vi "DataLog Read Log Time Range.vi"(0 "tag log directory":path, 5 "begin of range":dbl format="%<%H:%M:%S%2u\n%Y/%m/%d>T", 9 "end of range":dbl format="%<%H:%M:%S%2u\n%Y/%m/%d>T", 11 "error in (no error)":errorcluster) -> (4 "dup tag log directory":path, 6 "too many points?":bool, 8 "time range of points":T1[](array[typedef]) {"value" format="%.3e"; "time" format="%<%H:%M:%S%2u\n%Y/%m/%d>T"}, 15 "error out":errorcluster)   [LabVIEW 2012]
doc: "Read a range of points that covers the specified time range from a tag's log. The first returned point's time <= begin, the last returned point's time >= end. An exception to this rule occurs when the range begins before the oldest point in the log or ends after the last point in the log. In that case as much data as possible will be returned. If the range lies before the logged data, only the first point will be returned. If the range lies beyond the logged data, only the last point will be returned."
uses:
  typedefs/clusters/t_DataLog Point.ctl
  private/glb_DataLog MCVD.vi
  private/glb_DataLog Runtime Parameterisation.vi
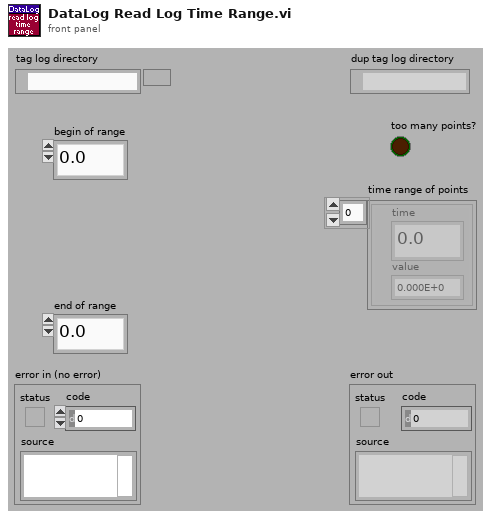
[diagram p1: front panel]
types:
  T1 = typedef "t_DataLog Point.ctl" = cluster{"time":dbl, "value":dbl}
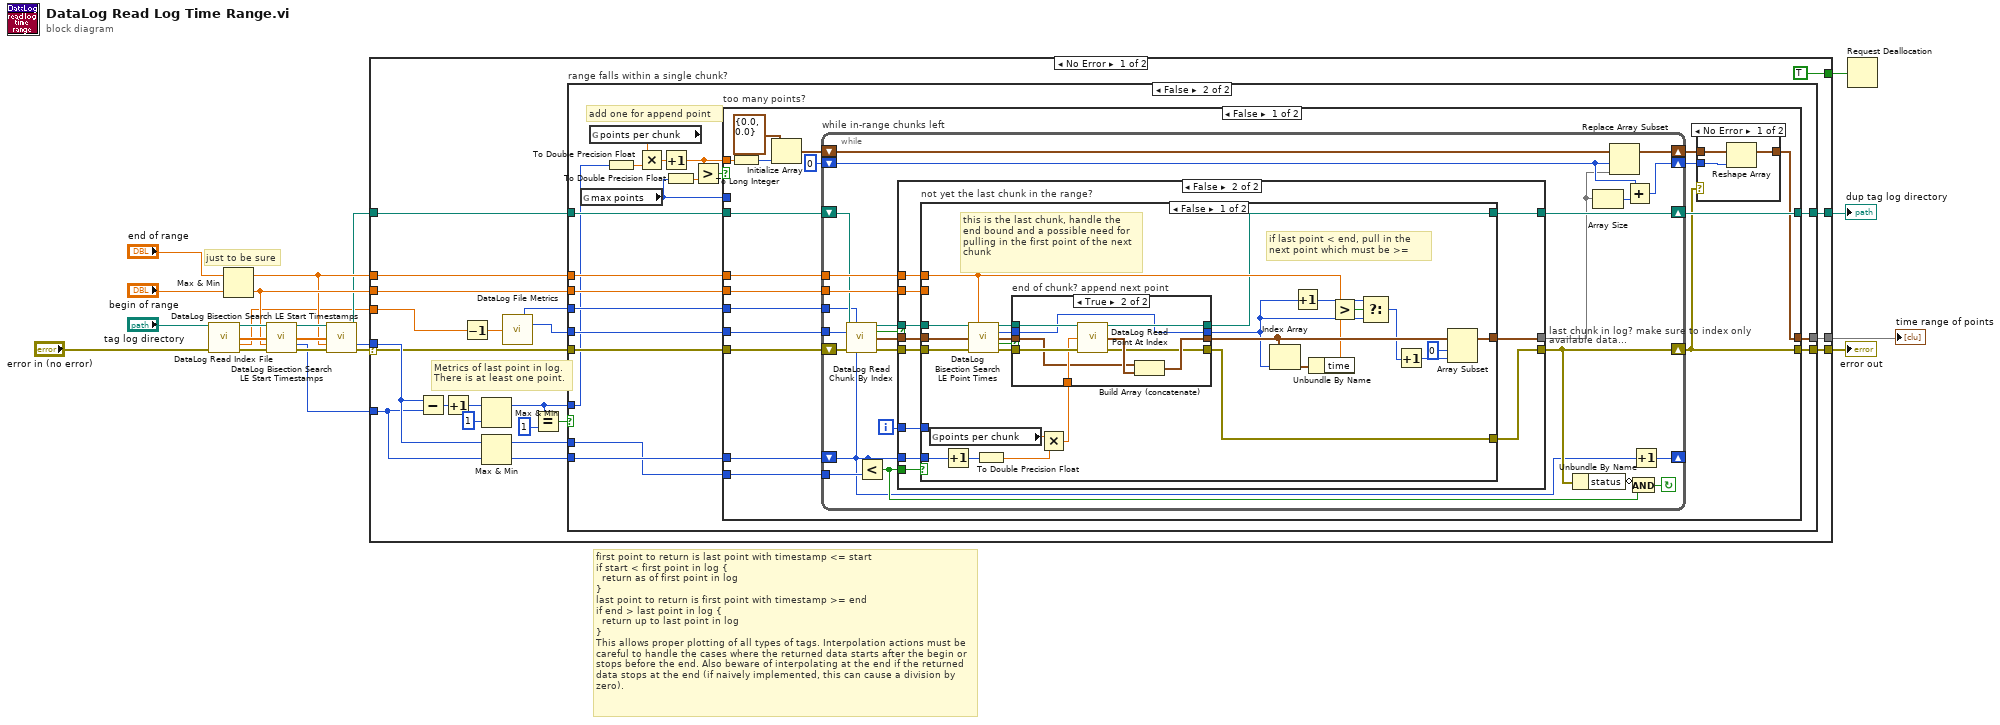
[diagram p0: block diagram]
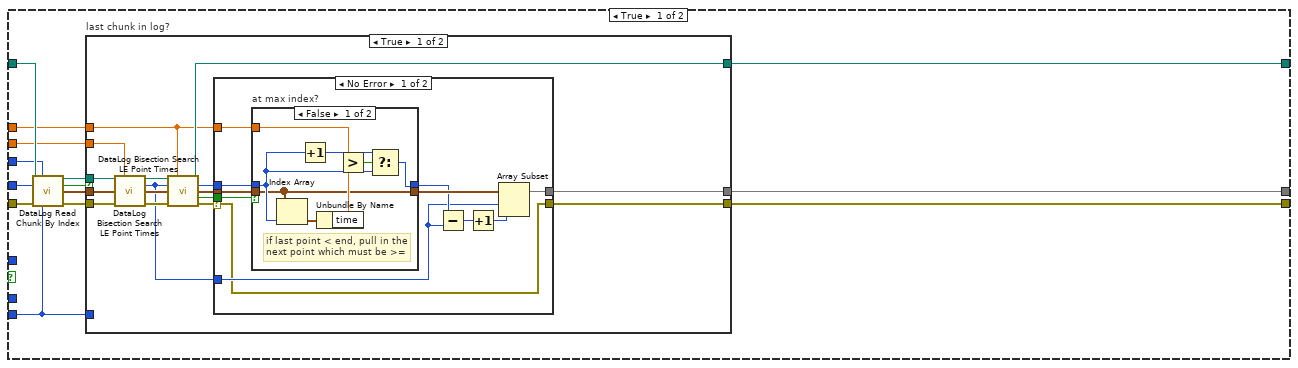
[diagram p2: hidden frame]
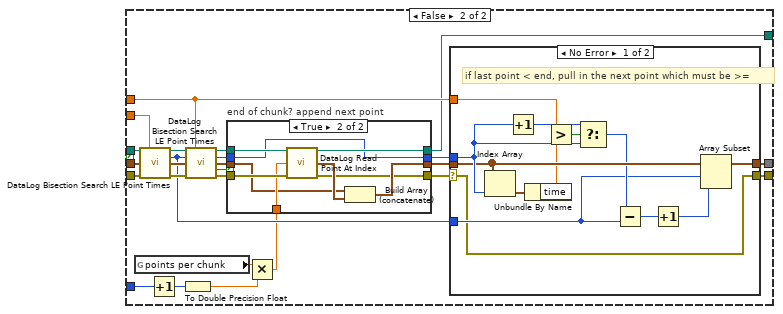
[diagram p5: hidden frame]
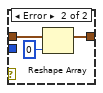
[diagram p8: hidden frame]
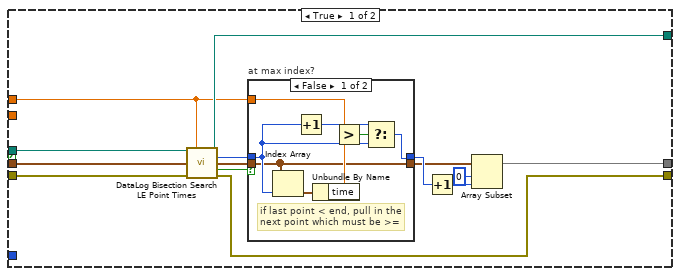
[diagram p9: hidden frame]
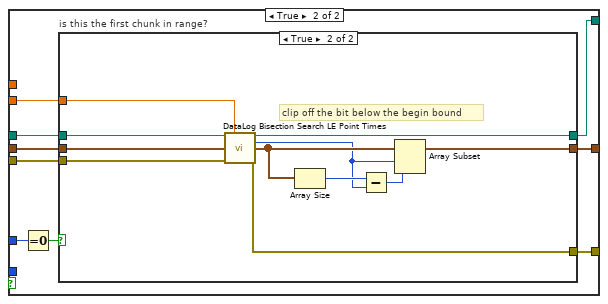
[diagram p12: hidden frame]
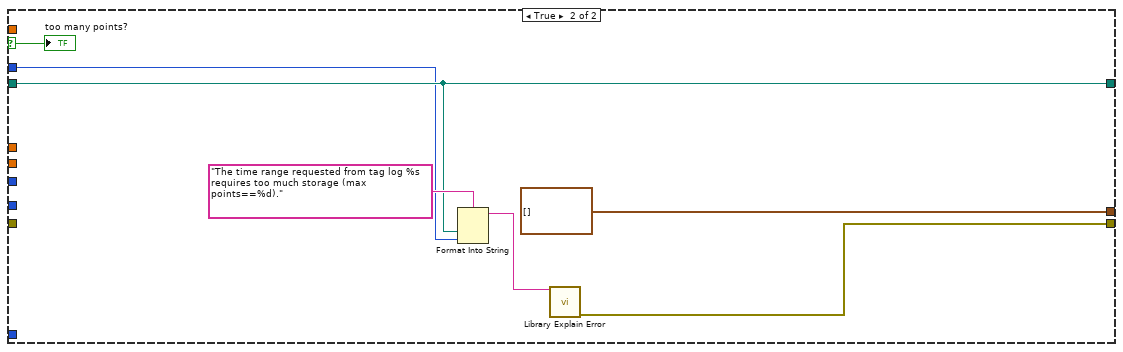
[diagram p14: hidden frame]
diagram:
  # "just to be sure"
  # "first point to return is last point with timestamp <= start\nif start < first point in log {\n  return as of first point in log\n}\nlast point to return is first point with timestamp >= end\nif end > last point in log {\n  return up to last point in log\n}\nThis allows proper plotting of all types of tags. Interpolation actions must be careful to handle the cases where the returned data starts after the begin or stops before the end. Also beware of interpolating at the end if the returned data stops at the end (if naively implemented, this can cause a division by zero)."
  n1 = call "DataLog Read Index File.vi"("tag log directory"="tag log directory", "error in (no error)"="error in (no error)") -> ("dup tag log directory"=w13:path, "chunk start timestamps"=w14:dbl[], "write index"=w4:dbl, "error out"=w12:errorcluster)  [unwired: 10 in]
  n2 = Max & Min(x="end of range", y="begin of range") -> (max(x,y)=w6:dbl, min(x,y)=w7:dbl)
  n3 = call "DataLog Bisection Search LE Start Timestamps.vi"("tag log directory"=w13, "chunk start timestamps"=w14, "search timestamp"=w7, "error in (no error)"=w12) -> ("dup tag log directory"=w11:path, "dup chunk start timestamps"=w10:dbl[], "nearest chunk index"=w3:i32, "error out"=w9:errorcluster)  [unwired: 8 in]
  n4 = call "DataLog Bisection Search LE Start Timestamps.vi"("tag log directory"=w11, "chunk start timestamps"=w10, "search timestamp"=w6, "error in (no error)"=w9) -> ("dup tag log directory"=w5:path, "nearest chunk index"=w8:i32, "error out"=w2:errorcluster)  [unwired: 8 in, 1 out]
  n5 = case shown="No Error" w2 {
    selector: w2 -> [w23 w320]
    tunnel: [w43 w320] -> w21
    tunnel: [w42 w321] -> w18
    tunnel: [w41 _] -> w17
    tunnel: w8 -> [w38 _]
    tunnel: w7 -> [w33 _]
    tunnel: w6 -> [w32 _]
    tunnel: w5 -> [w30 w321]
    tunnel: w4 -> [w27 _]
    tunnel: w3 -> [w24 _]
    tunnel: [TRUE _] -> w1
    frame No Error {
      # "Metrics of last point in log.\nThere is at least one point."
      n6 = Subtract(x=w38, y=w24) -> (x-y=w40:i32)
      n7 = Increment(x=w40) -> (x+1=w34:i32)
      n8 = Decrement(x=w27) -> (x-1=w28:dbl)
      n9 = Max & Min(x=w34, y=1) -> (max(x,y)=w25:i32)  [unwired: 1 out]
      n10 = Max & Min(x=w38, y=w24) -> (max(x,y)=w31:i32, min(x,y)=w37:i32)
      n11 = call "DataLog File Metrics.vi"("point index"=w28) -> ("index in chunk"=w26:i32, "chunk index"=w29:i32)  [unwired: 9 in, 4 out]
      n12 = Equal?(x=w25, y=1) -> (x = y?=w35:bool)
      n13 = case "range falls within a single chunk?" shown="False" w35 {
        tunnel: w30 -> [w57 w161]
        tunnel: w23 -> [w56 w159]
        tunnel: w37 -> [w45 w162]
        tunnel: w33 -> [w51 w166]
        tunnel: w32 -> [w50 w165]
        tunnel: [w52 w154] -> w43
        tunnel: [w49 w160] -> w42
        tunnel: w31 -> [_ w155]
        tunnel: w29 -> [w46 w163]
        tunnel: w26 -> [w44 w164]
        tunnel: [w48 w153] -> w41
        tunnel: w25 -> [_ w158]
        frame True {
          n14 = call "DataLog Read Chunk By Index.vi"("tag log directory"=w57, "index in last chunk"=w44, "index of last chunk"=w46, "error in (no error)"=w56, "chunk index"=w45) -> ("dup tag log directory"=w53:path, "last chunk in log?"=w47:bool, "chunk of points"=w54:T1[], "error out"=w55:errorcluster)  [unwired: 7 in]
          n15 = case "last chunk in log?" shown="True" w47 {
            tunnel: w55 -> [w73 w120]
            tunnel: w54 -> [w72 w119]
            tunnel: w53 -> [w68 w115]
            tunnel: [w62 w111] -> w52
            tunnel: w51 -> [w66 w114]
            tunnel: w50 -> [w59 w112]
            tunnel: [w65 w102] -> w49
            tunnel: [w63 w110] -> w48
            tunnel: w45 -> [_ w96]
            frame True {
              n16 = call "DataLog Bisection Search LE Point Times.vi"("tag log directory"=w68, "search timestamp"=w66, "points"=w72, "error in (no error)"=w73) -> ("dup tag log directory"=w69:path, "index"=w58:i32, "dup points"=w71:T1[], "error out"=w70:errorcluster)  [unwired: 7 in, 1 out]
              n17 = call "DataLog Bisection Search LE Point Times.vi"("tag log directory"=w69, "search timestamp"=w59, "min index (0)"=w58, "points"=w71, "error in (no error)"=w70) -> ("dup tag log directory"=w65:path, "index"=w61:i32, "dup points"=w67:T1[], "at max?"=w60:bool, "error out"=w64:errorcluster)  [unwired: 6 in]
              n18 = case shown="No Error" w64 {
                selector: w64 -> [w74 w95]
                tunnel: w67 -> [w82 _]
                tunnel: [w79 _] -> w63
                tunnel: [w74 w95] -> w62
                tunnel: w61 -> [w83 _]
                tunnel: w60 -> [w84 _]
                tunnel: w59 -> [w81 _]
                tunnel: w58 -> [w77 _]
                frame No Error {
                  n19 = case "at max index?" shown="False" w84 {
                    tunnel: w83 -> [w87 w94]
                    tunnel: [w86 w94] -> w78
                    tunnel: [w85 w93] -> w80
                    tunnel: w82 -> [w85 w93]
                    tunnel: w81 -> [w91 _]
                    frame False {
                      # "if last point < end, pull in the next point which must be >="
                      n20 = Index Array(array=w85, index=w87) -> (element=w92:T1)
                      n21 = Increment(x=w87) -> (x+1=w88:i32)
                      n22 = Unbundle By Name(w92) -> ("time"=w90:dbl)
                      n23 = Greater?(x=w91, y=w90) -> (0:w89:bool)
                      n24 = Select(t=w88, s=w89, f=w87) -> (s? t:f=w86:i32)
                    }
                    frame True {
                    }
                  }
                  n25 = Subtract(x=w78, y=w77) -> (x-y=w76:i32)
                  n26 = Increment(x=w76) -> (x+1=w75:i32)
                  n27 = Array Subset(array=w80, index=w77, length=w75) -> (w79:T1[])
                }
                frame Error {
                }
              }
            }
            frame False {
              n28 = global read "glb_DataLog MCVD.vi" "points per chunk"() -> (w100:dbl)
              n29 = call "DataLog Bisection Search LE Point Times.vi"("tag log directory"=w115, "search timestamp"=w114, "points"=w119, "error in (no error)"=w120) -> ("dup tag log directory"=w116:path, "index"=w113:i32, "dup points"=w118:T1[], "error out"=w117:errorcluster)  [unwired: 7 in, 1 out]
              n30 = Increment(x=w96) -> (x+1=w97:i32)
              n31 = To Double Precision Float(number=w97) -> (double precision float=w99:dbl)
              n32 = call "DataLog Bisection Search LE Point Times.vi"("tag log directory"=w116, "search timestamp"=w112, "min index (0)"=w113, "points"=w118, "error in (no error)"=w117) -> ("dup tag log directory"=w107:path, "index"=w103:i32, "dup points"=w106:T1[], "at max?"=w109:bool, "error out"=w108:errorcluster)  [unwired: 6 in]
              n33 = Multiply(x=w100, y=w99) -> (x*y=w98:dbl)
              n34 = case "end of chunk? append next point" shown="True" w109 {
                tunnel: w108 -> [w121 w133]
                tunnel: w107 -> [w122 w131]
                tunnel: [w124 w128] -> w105
                tunnel: w106 -> [w124 w129]
                tunnel: w103 -> [w123 w125]
                tunnel: [w123 w125] -> w104
                tunnel: [w122 w127] -> w102
                tunnel: [w121 w126] -> w101
                tunnel: w98 -> [_ w132]
                frame False {
                }
                frame True {
                  n35 = call "DataLog Read Point At Index.vi"("tag log directory"=w131, "log index"=w132, "error in (no error)"=w133) -> ("dup tag log directory"=w127:path, "point"=w130:T1, "error out"=w126:errorcluster)  [unwired: 10 in]
                  n36 = Build Array (concatenate)(w129, w130) -> (w128:T1[])
                }
              }
              n37 = case shown="No Error" w101 {
                selector: w101 -> [w134 w147]
                tunnel: w105 -> [w145 _]
                tunnel: [w143 _] -> w110
                tunnel: [w134 w147] -> w111
                tunnel: w104 -> [w146 _]
                tunnel: w112 -> [w144 _]
                tunnel: w113 -> [w141 _]
                frame No Error {
                  # "if last point < end, pull in the next point which must be >="
                  n38 = Index Array(array=w145, index=w146) -> (element=w140:T1)
                  n39 = Increment(x=w146) -> (x+1=w137:i32)
                  n40 = Unbundle By Name(w140) -> ("time"=w139:dbl)
                  n41 = Greater?(x=w144, y=w139) -> (0:w138:bool)
                  n42 = Select(t=w137, s=w138, f=w146) -> (s? t:f=w142:i32)
                  n43 = Subtract(x=w142, y=w141) -> (x-y=w136:i32)
                  n44 = Increment(x=w136) -> (x+1=w135:i32)
                  n45 = Array Subset(array=w145, index=w141, length=w135) -> (w143:T1[])
                }
                frame Error {
                }
              }
            }
          }
        }
        frame False {
          # "add one for append point"
          n46 = global read "glb_DataLog Runtime Parameterisation.vi" "max points"() -> (w148:i32)
          n47 = global read "glb_DataLog MCVD.vi" "points per chunk"() -> (w156:dbl)
          n48 = To Double Precision Float(number=w158) -> (double precision float=w157:dbl)
          n49 = Multiply(x=w156, y=w157) -> (x*y=w151:dbl)
          n50 = Increment(x=w151) -> (x+1=w150:dbl)
          n51 = To Double Precision Float(number=w148) -> (double precision float=w149:dbl)
          n52 = Greater?(x=w150, y=w149) -> (0:w152:bool)
          n53 = case "too many points?" shown="False" w152 {
            selector: w152 -> [_ w313]
            tunnel: w166 -> [w184 _]
            tunnel: w165 -> [w183 _]
            tunnel: w164 -> [w182 _]
            tunnel: w163 -> [w181 _]
            tunnel: w162 -> [w180 _]
            tunnel: w161 -> [w179 w315]
            tunnel: [w178 w315] -> w160
            tunnel: w159 -> [w177 _]
            tunnel: [w169 T1[] []] -> w153
            tunnel: [w168 w318] -> w154
            tunnel: w155 -> [w176 _]
            tunnel: w150 -> [w175 _]
            tunnel: w148 -> [_ w314]
            frame False {
              n54 = To Long Integer(number=w175) -> (32bit integer=w174:i32)
              n55 = Initialize Array(T1 {"time"=0.0, "value"=0.0} ("point"), w174) -> (w167:T1[])
              n56 = while "while in-range chunks left" {
                tunnel: w184 -> [w212]
                tunnel: w183 -> [w211]
                tunnel: w182 -> [w195]
                tunnel: w181 -> [w193]
                shift-right: [w207] -> _
                shift-left: w180 -> [w194]
                shift-right: [w209] -> w178
                shift-left: w179 -> [w210]
                shift-right: [w196] -> w171
                shift-left: w167 -> [w203]
                shift-right: [w205] -> w168
                shift-left: w177 -> [w208]
                tunnel: w176 -> [w206]
                shift-right: [w201] -> w170
                shift-left: 0 -> [w202]
                i -> [w198]
                stop <- w204 continue-if-true
                n57 = call "DataLog Read Chunk By Index.vi"("tag log directory"=w210, "index in last chunk"=w195, "index of last chunk"=w193, "error in (no error)"=w208, "chunk index"=w194) -> ("dup tag log directory"=w213:path, "last chunk in log?"=w192:bool, "chunk of points"=w214:T1[], "error out"=w215:errorcluster)  [unwired: 7 in]
                n58 = Less?(x=w194, y=w206) -> (x < y?=w199:bool)
                n59 = case "last chunk in log? make sure to index only available data..." shown="False" w192 {
                  tunnel: w215 -> [w221 w244]
                  tunnel: w214 -> [w222 w245]
                  tunnel: w213 -> [w223 w243]
                  tunnel: [w216 w249] -> w205
                  tunnel: w212 -> [_ w240]
                  tunnel: w211 -> [w224 w250]
                  tunnel: [w228 w247] -> w209
                  tunnel: [w227 w248] -> w191
                  tunnel: w194 -> [_ w246]
                  tunnel: w199 -> [_ w242]
                  tunnel: w198 -> [_ w241]
                  frame True {
                    n60 = call "DataLog Bisection Search LE Point Times.vi"("tag log directory"=w223, "search timestamp"=w224, "points"=w222, "error in (no error)"=w221) -> ("dup tag log directory"=w228:path, "index"=w226:i32, "dup points"=w229:T1[], "at max?"=w225:bool, "error out"=w216:errorcluster)  [unwired: 7 in]
                    n61 = case "at max index?" shown="False" w225 {
                      tunnel: w226 -> [w232 w239]
                      tunnel: [w231 w239] -> w220
                      tunnel: [w230 w238] -> w219
                      tunnel: w229 -> [w230 w238]
                      tunnel: w224 -> [w236 _]
                      frame False {
                        # "if last point < end, pull in the next point which must be >="
                        n62 = Index Array(array=w230, index=w232) -> (element=w237:T1)
                        n63 = Increment(x=w232) -> (x+1=w233:i32)
                        n64 = Unbundle By Name(w237) -> ("time"=w235:dbl)
                        n65 = Greater?(x=w236, y=w235) -> (0:w234:bool)
                        n66 = Select(t=w233, s=w234, f=w232) -> (s? t:f=w231:i32)
                      }
                      frame True {
                      }
                    }
                    n67 = Increment(x=w220) -> (x+1=w218:i32)
                    n68 = Array Subset(array=w219, index=0, length=w218) -> (w227:T1[])
                  }
                  frame False {
                    n69 = case "not yet the last chunk in the range?" shown="False" w242 {
                      tunnel: w250 -> [w276 _]
                      tunnel: [w275 w294] -> w249
                      tunnel: [w274 w295] -> w248
                      tunnel: [w266 w291] -> w247
                      tunnel: w246 -> [w261 _]
                      tunnel: w245 -> [w260 w296]
                      tunnel: w244 -> [w259 w293]
                      tunnel: w243 -> [w258 w292]
                      tunnel: w241 -> [_ w298]
                      tunnel: w240 -> [_ w290]
                      frame False {
                        # "if last point < end, pull in the next point which must be >="
                        # "this is the last chunk, handle the\nend bound and a possible need for\npulling in the first point of the next\nchunk"
                        n70 = global read "glb_DataLog MCVD.vi" "points per chunk"() -> (w265:dbl)
                        n71 = Increment(x=w261) -> (x+1=w262:i32)
                        n72 = call "DataLog Bisection Search LE Point Times.vi"("tag log directory"=w258, "search timestamp"=w276, "points"=w260, "error in (no error)"=w259) -> ("dup tag log directory"=w271:path, "index"=w267:i32, "dup points"=w270:T1[], "at max?"=w273:bool, "error out"=w272:errorcluster)  [unwired: 7 in]
                        n73 = To Double Precision Float(number=w262) -> (double precision float=w264:dbl)
                        n74 = Multiply(x=w265, y=w264) -> (x*y=w263:dbl)
                        n75 = case "end of chunk? append next point" shown="True" w273 {
                          tunnel: w272 -> [w277 w289]
                          tunnel: w271 -> [w278 w287]
                          tunnel: [w280 w284] -> w269
                          tunnel: w270 -> [w280 w285]
                          tunnel: w267 -> [w279 w281]
                          tunnel: [w279 w281] -> w268
                          tunnel: [w278 w283] -> w266
                          tunnel: [w277 w282] -> w275
                          tunnel: w263 -> [_ w288]
                          frame False {
                          }
                          frame True {
                            n76 = call "DataLog Read Point At Index.vi"("tag log directory"=w287, "log index"=w288, "error in (no error)"=w289) -> ("dup tag log directory"=w283:path, "point"=w286:T1, "error out"=w282:errorcluster)  [unwired: 10 in]
                            n77 = Build Array (concatenate)(w285, w286) -> (w284:T1[])
                          }
                        }
                        n78 = Index Array(array=w269, index=w268) -> (element=w257:T1)
                        n79 = Increment(x=w268) -> (x+1=w254:i32)
                        n80 = Unbundle By Name(w257) -> ("time"=w256:dbl)
                        n81 = Greater?(x=w276, y=w256) -> (0:w255:bool)
                        n82 = Select(t=w254, s=w255, f=w268) -> (s? t:f=w252:i32)
                        n83 = Increment(x=w252) -> (x+1=w253:i32)
                        n84 = Array Subset(array=w269, index=0, length=w253) -> (w274:T1[])
                      }
                      frame True {
                        n85 = Equal To 0?(x=w298) -> (x = 0?=w297:bool)
                        n86 = case "is this the first chunk in range?" shown="True" w297 {
                          tunnel: w296 -> [w301 w309]
                          tunnel: [w301 w307] -> w295
                          tunnel: [w300 w306] -> w294
                          tunnel: w293 -> [w300 w310]
                          tunnel: w292 -> [w299 w312]
                          tunnel: [w299 w311] -> w291
                          tunnel: w290 -> [_ w308]
                          frame False {
                            # "any intermediate chunk is appended whole"
                          }
                          frame True {
                            # "clip off the bit below the begin bound"
                            n87 = call "DataLog Bisection Search LE Point Times.vi"("tag log directory"=w312, "search timestamp"=w308, "points"=w309, "error in (no error)"=w310) -> ("dup tag log directory"=w311:path, "index"=w303:i32, "dup points"=w305:T1[], "error out"=w306:errorcluster)  [unwired: 7 in, 1 out]
                            n88 = Array Size(array=w305) -> (size(s)=w304:i32)
                            n89 = Subtract(x=w304, y=w303) -> (x-y=w302:i32)
                            n90 = Array Subset(array=w305, index=w303, length=w302) -> (w307:T1[])
                          }
                        }
                      }
                    }
                  }
                }
                n91 = Unbundle By Name(w205) -> ("status"=w197:bool)
                n92 = Array Size(array=w191) -> (size(s)=w200:i32)
                n93 = Replace Array Subset(array=w203, new element=w191, index=w202) -> (w196:T1[])
                n94 = Add(x=w202, y=w200) -> (x+y=w201:i32)
                n95 = Increment(x=w194) -> (x+1=w207:i32)
                n96 = Compound Arithmetic op=AND(invert w197, w199) -> (w204:bool)
              }
              n97 = case shown="No Error" w168 {
                tunnel: w171 -> [w187 w190]
                tunnel: w170 -> [w185 _]
                tunnel: [w186 w189] -> w169
                frame No Error {
                  n98 = Reshape Array(w187, w185) -> (w186:T1[])
                }
                frame Error {
                  n99 = Reshape Array(w190, 0 ("dimension size")) -> (w189:T1[])
                }
              }
            }
            frame True {
              n100 = Format Into String(format string="The time range requested from tag log %s requires too much storage (max points==%d).", w315, w314) -> (resulting string=w316:string)  [unwired: 2 in, 1 out]
              n101 = call "Library Explain Error.vi"("explanation prefix (none)"=w316) -> ("explained error"=w318:errorcluster)  [unwired: 14 in]
              "too many points?" <- w313
            }
          }
        }
      }
    }
    frame Error {
    }
  }
  "error out" <- w21
  "dup tag log directory" <- w18
  "time range of points" <- w17
  n102 = Request Deallocation(w1) -> ()
